vi "FGV_save_time.vi"(7 "Action":T2=enum."Reset", 8 "error in (no error)":errorcluster, 11 "DateTime":T1={"date"="30/01/2019", "time"="16:37:13"}) -> (0 "error out":errorcluster, 3 "DateTime out":T1)   [LabVIEW 2018]
uses:
  Controls/Date Time cluster.ctl
  Controls/FGV_savetime_action.ctl
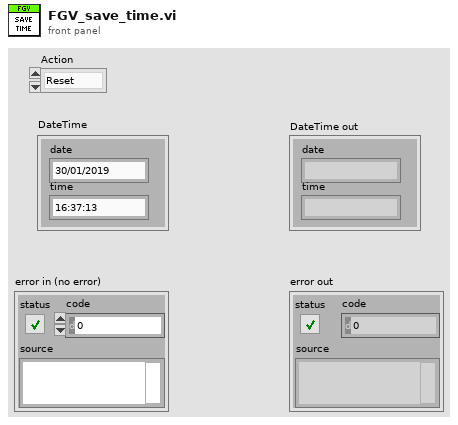
[diagram p1: front panel]
types:
  T1 = typedef "Date Time cluster.ctl" = cluster{"date":string, "time":string}
  T2 = typedef "FGV_savetime_action.ctl" = enum16{"Save", "Read", "Reset"}
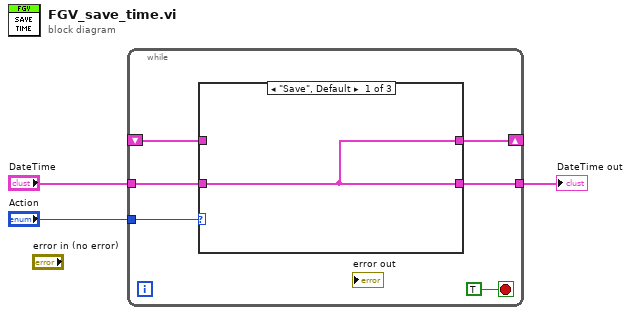
[diagram p0: block diagram]
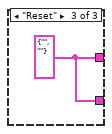
[diagram p3: hidden frame]
diagram:
  n1 = while {
    tunnel: "Action" -> [w8]
    shift-right: [w5] -> _
    shift-left: _ -> [w6]
    tunnel: [w7] -> w2
    tunnel: "DateTime" -> [w4]
    stop <- TRUE stop-if-true
    n2 = case shown="\"Save\", Default" w8 {
      tunnel: [w10 w11 w12] -> w7
      tunnel: w6 -> [_ w11 _]
      tunnel: [w10 w11 w12] -> w5
      tunnel: w4 -> [w10 _ _]
      frame "Save", Default {
      }
      frame "Read" {
      }
      frame "Reset" {
        w12 = T1 {"date"="", "time"=""} ("DateTime")
      }
    }
  }
  "DateTime out" <- w2
